vi "Single Command.vi"(8 "error in (no error)":errorcluster, 9 "Variant (Cluster, Array,..)":variant, 10 "SQL (Single Command)":string, 11 "PQ Connection in":refnum<class "PQ Connection.lvclass">) -> (0 "error out":errorcluster, 1 "First Result with Rows returned":refnum<class "PQ Result.lvclass">, 2 "Number of Rows":i32, 3 "PQ Connection out":refnum<class "PQ Connection.lvclass">)   [LabVIEW 2015, in "PQ Connection.lvclass"]
uses:
  PQ Connection.lvclass
  Result/PQ Result.lvclass
  <vilib>/Utility/Data Type/NI_Data Type.lvlib
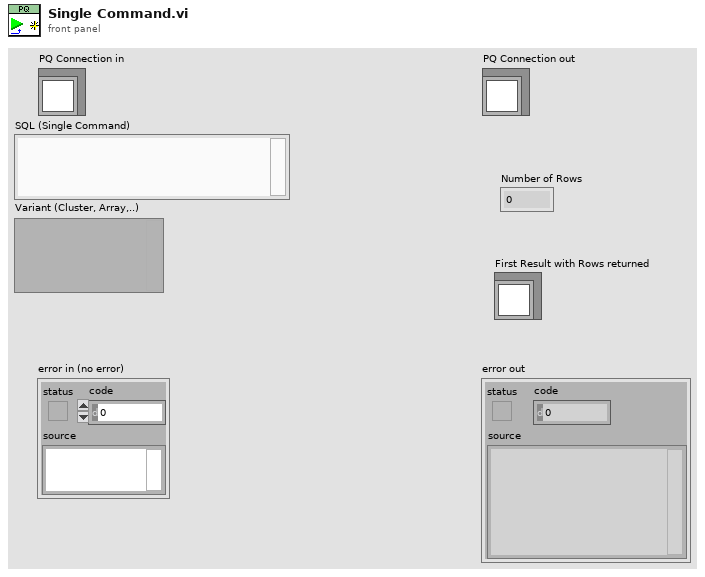
[diagram p1: front panel]
types:
  T1 = typedef "NI_Data Type.lvlib/Data Type.ctl" = enum8{"Invalid Type", "Void", "I8", "I16", "I32", "I64", "U8", "U16", "U32", "U64", "Single Float", "Double Float", "Extended Float", "Single Complex", "Double Complex", "Extended Complex", "Enum U8", "Enum U16", "Enum U32", "Enum U64", "Single Float With Unit", "Double Float With Unit", "Extended Float With Unit", "Single Complex with Unit", "Double Complex with Unit", "Extended Complex with Unit", "Boolean", "String", "Path", "Picture", "Tag", "Array", "Cluster", "Variant", "LV Variant", "Waveform", "Timestamp", "Digital Waveform", "Digital Data", "ExpressData", "Refnum", "External Data", "VI", "Poly VI", "LabVIEW Class Instance", "Fixed Point"}
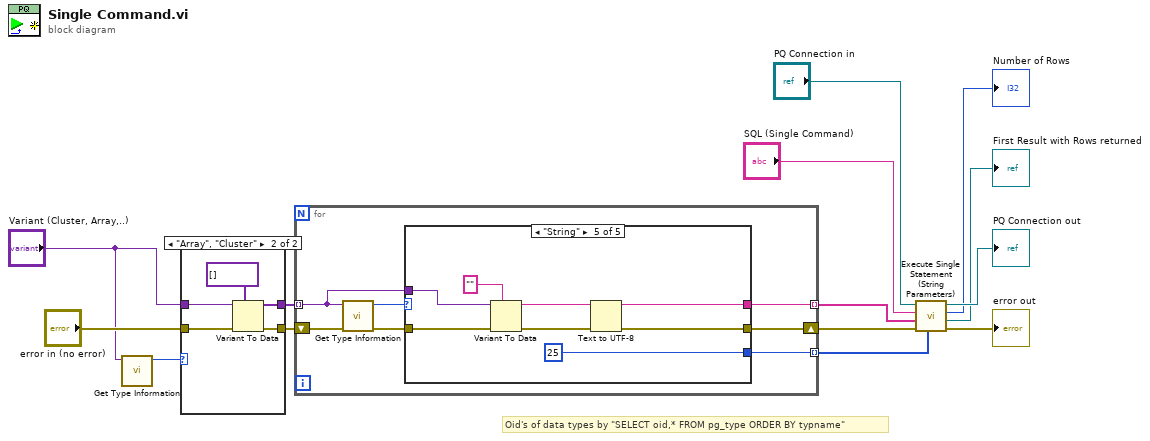
[diagram p0: block diagram]
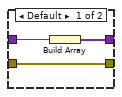
[diagram p2: hidden frame]
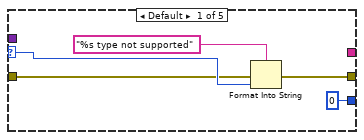
[diagram p3: hidden frame]
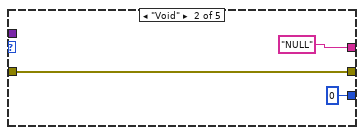
[diagram p4: hidden frame]
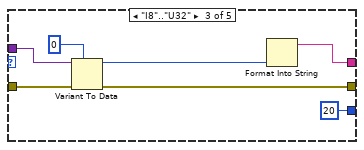
[diagram p5: hidden frame]
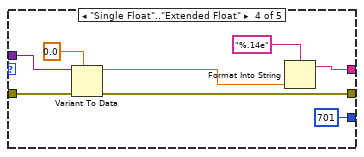
[diagram p6: hidden frame]
diagram:
  # "Oid's of data types by \"SELECT oid,* FROM pg_type ORDER BY typname\""
  n1 = call <vilib>:"Get Type Information.vi"("Variant"="Variant (Cluster, Array,..)") -> ("Type"=w2:T1)  [unwired: 6 in, 4 out]
  n2 = case shown="\"Array\", \"Cluster\"" w2 {
    tunnel: [w16 w21] -> w14
    tunnel: [w15 w20] -> w13
    tunnel: "error in (no error)" -> [w15 w19]
    tunnel: "Variant (Cluster, Array,..)" -> [w17 w18]
    frame Default {
      n3 = Build Array(w17) -> (w16:variant[])
    }
    frame "Array", "Cluster" {
      n4 = Variant To Data(error in=w19, type=variant[] [], Variant=w18) -> (data=w21:variant[], error out=w20:errorcluster)
    }
  }
  n5 = for {
    tunnel: w14 -> [w28] mode=indexing
    tunnel: [w27] -> w7 mode=indexing
    shift-right: [w24] -> w8
    shift-left: w13 -> [w26]
    tunnel: [w23] -> w1 mode=indexing
    n6 = call <vilib>:"Get Type Information.vi"("error in (no error)"=w26, "Variant"=w28) -> ("error out"=w25:errorcluster, "Type"=w29:T1)  [unwired: 5 in, 3 out]
    n7 = case shown="\"String\"" w29 {
      selector: w29 -> [w34 _ _ _ _]
      tunnel: w28 -> [_ _ w44 w52 w60]
      tunnel: [_ "NULL" w41 w49 w55] -> w27
      tunnel: w25 -> [w32 w36 w40 w47 w58]
      tunnel: [w31 w36 w39 w46 w53] -> w24
      tunnel: [0 0 20 701 25] -> w23
      frame Default {
        n8 = Format Into String(format string="%s type not supported", error in=w32, w34) -> (error out=w31:errorcluster)  [unwired: 1 in, 1 out]
      }
      frame "Void" {
      }
      frame "I8".."U32" {
        n9 = Variant To Data(error in=w40, type=i64 0, Variant=w44) -> (data=w42:i64, error out=w39:errorcluster)
        n10 = Format Into String(w42) -> (resulting string=w41:string)  [unwired: 3 in, 1 out]
      }
      frame "Single Float".."Extended Float" {
        n11 = Variant To Data(error in=w47, type=0.0, Variant=w52) -> (data=w50:dbl, error out=w46:errorcluster)
        n12 = Format Into String(format string="%.14e", w50) -> (resulting string=w49:string)  [unwired: 2 in, 1 out]
      }
      frame "String" {
        n13 = Variant To Data(error in=w58, type="", Variant=w60) -> (data=w56:string, error out=w54:errorcluster)
        n14 = Text to UTF-8(8:w54, 11:w56) -> (0:w53:errorcluster, 3:w55:string)  [unwired: 1 in]
      }
    }
  }
  n15 = call "Execute Single Statement (String Parameters).vi"("Oids"=w1, "error in (no error)"=w8, "Parameters"=w7, "SQL (Single Command)"="SQL (Single Command)", "PQ Connection in"="PQ Connection in") -> ("error out"=→"error out":errorcluster, "First Result with Rows returned"=→"First Result with Rows returned":refnum<class "PQ Result.lvclass">, "Number of Rows"=→"Number of Rows":i32, "PQ Connection out"=→"PQ Connection out":refnum<class "PQ Connection.lvclass">)  [unwired: 3 in]
